vi "PI_sandbox.vi"() -> ()   [LabVIEW 2013]
uses:
  <vilib>/addons/control/pid/pid.llb/PID (DBL).vi
  <vilib>/addons/control/pid/NI_PID_pid.lvlib
  <vilib>/ptbypt/NI_PtbyPt.lvlib
panel:
  in  "stop":bool
  out "Waveform Graph":dbl[][](graph)
  in  "Min":dbl=1.0 format="%#_13g"
  in  "Max":dbl=1.0 format="%#_13g"
  in  "Ki":dbl=1.0 format="%#_13g"
  in  "Kp":dbl=1.0 format="%#_13g"
  in  "dt":dbl=1.0 format="%#_13g"
  # "NI\nAlternate\nInput"
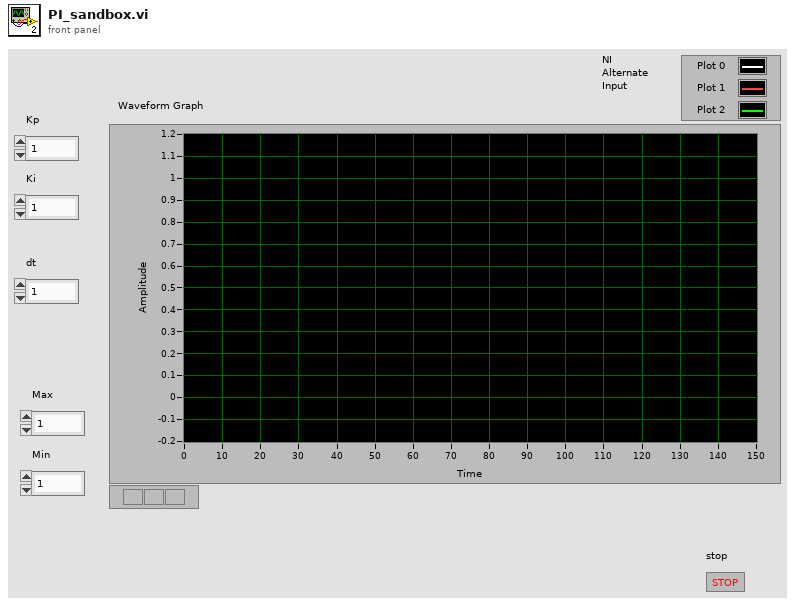
[diagram p1: front panel]
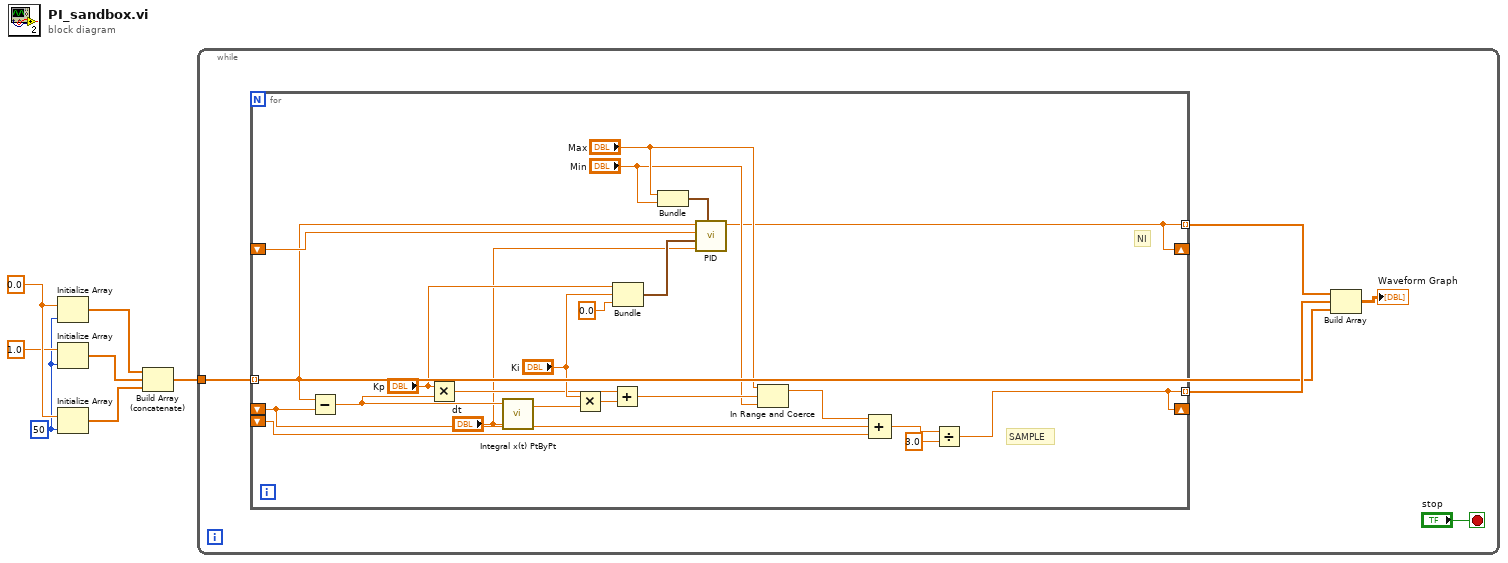
[diagram p0: block diagram]
diagram:
  w3 = 50 ("dimension size")
  w5 = 0.0
  n1 = Initialize Array(w5, w3) -> (w7:dbl[])
  n2 = Initialize Array(1.0, w3) -> (w6:dbl[])
  n3 = Initialize Array(w5, w3) -> (w1:dbl[])
  n4 = Build Array (concatenate)(w7, w6, w1) -> (w2:dbl[])
  n5 = while {
    tunnel: w2 -> [w8]
    stop <- "stop" stop-if-true
    n6 = for {
      tunnel: w8 -> [w21] mode=indexing
      tunnel: [w20] -> w12 mode=indexing
      tunnel: [w13] -> w10 mode=indexing
      shift-right: [w13] -> _
      shift-left: _ -> [w18]
      shift-right: [w20] -> _
      shift-left: _ -> [w25]
      shift-left: _ -> [w17]
      # "SAMPLE"
      # "NI"
      n7 = Subtract(x=w21, y=w18) -> (x-y=w22:dbl)
      n8 = Multiply(x="Kp", y=w22) -> (x*y=w23:dbl)
      n9 = call <vilib>:"Integral x(t) PtByPt.vi"("dt"="dt", "x"=w22) -> ("integral x(t)"=w30:dbl)  [unwired: 2 in, 1 out]
      n10 = Multiply(x="Ki", y=w30) -> (x*y=w29:dbl)
      n11 = Add(x=w23, y=w29) -> (x+y=w28:dbl)
      n12 = Bundle("Kp"="Kp", "Ki"="Ki", 0.0) -> (w33:cluster{"Kp":dbl, "Ki":dbl, dbl})  [unwired: 1 in]
      n13 = Bundle("Max"="Max", "Min"="Min") -> (w32:cluster{"Max":dbl, "Min":dbl})  [unwired: 1 in]
      n14 = call-poly <vilib>:"PID.vi"("output range"=w32, "dt (s)"="dt", "PID gains"=w33, "process variable"=w25, "setpoint"=w21) -> ("output"=w20:dbl)  [unwired: 5 in, 1 out]
      n15 = In Range and Coerce(upper limit="Max", x=w28, lower limit="Min") -> (coerced(x)=w16:dbl)  [unwired: 1 out]
      n16 = Compound Arithmetic op=ADD(w16, w18, w17) -> (w15:dbl)
      n17 = Divide(x=w15, y=3.0) -> (x/y=w13:dbl)
    }
    n18 = Build Array(w12, w10, w8) -> (→"Waveform Graph":dbl[][])
  }
